vi "Create Fast Draw Object.vi"(6 "Actual Transform In":T1, 8 "error in (no error)":errorcluster, 9 "Multiplot Representation In":T3, 10 "3D Contour in":refnum<class "3D Contour.lvclass">, 11 "Plot Object In":refnum<vi>) -> (0 "error out":errorcluster, 1 "Multiplot Representation In":T3, 2 "3D Contour out":refnum<class "3D Contour.lvclass">, 3 "Plot Object Out":refnum<vi>, 4 "Actual Transform Out":T1)   [LabVIEW 2020, in "3D Contour.lvclass"]
uses:
  <vilib>/Math Plots/3D Math Plots/3D Contour/3D Contour/3D Contour.lvclass
  <vilib>/Math Plots/3D Math Plots/3D Plot/3D Plot/Typedef/Multiplot Representation.ctl
  <vilib>/Math Plots/3D Math Plots/3D Plot/3D Plot/Typedef/Plot Representation.ctl
  <vilib>/Math Plots/3D Math Plots/3D Plot/3D Plot/Typedef/Range Clusters.ctl
  <vilib>/Math Plots/3D Math Plots/3D Plot/3D Plot/Typedef/Mesh Data.ctl
  <vilib>/Math Plots/3D Math Plots/3D Plot/3D Plot/Typedef/Actual Transform.ctl
  <vilib>/Math Plots/3D Math Plots/3D Contour/3D Contour/3D Contour.lvclass/3D Contour.ctl
  <vilib>/Math Plots/3D Math Plots/3D Plot/3D Plot/3D Plot.lvclass
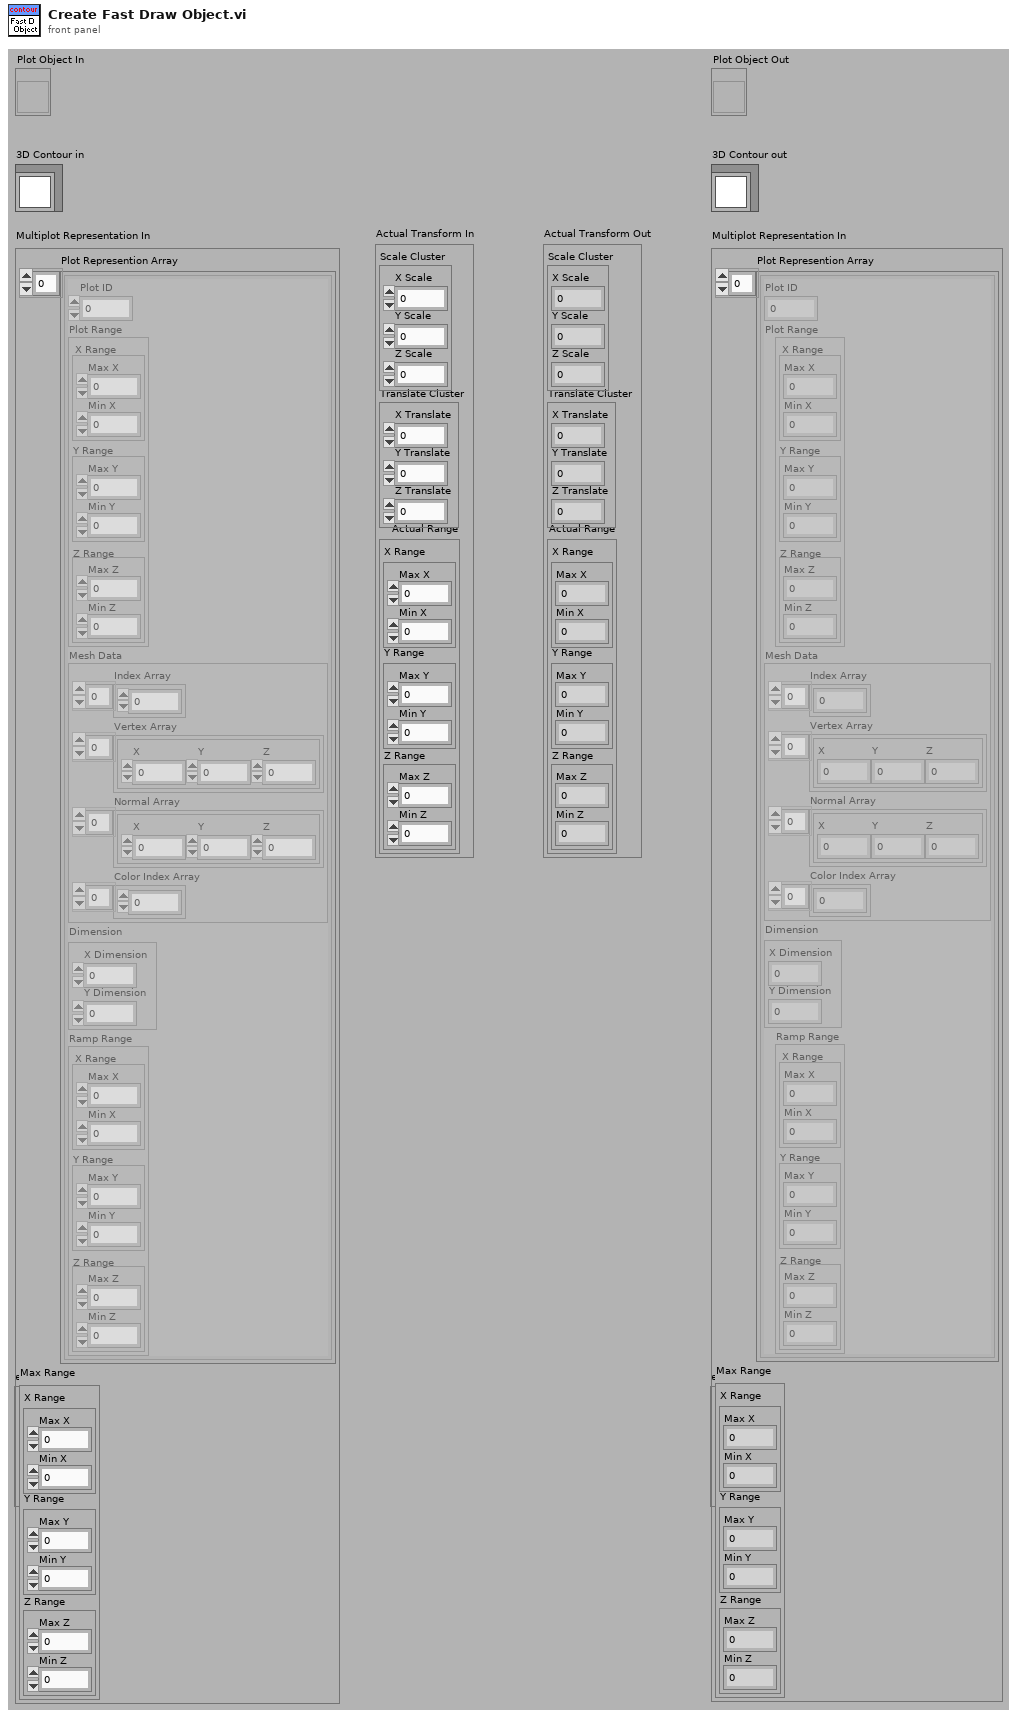
[diagram p1: front panel]
types:
  T1 = typedef "3D Plot.lvclass/Actual Transform.ctl" = cluster{"Scale Cluster":cluster{"X Scale":sgl, "Y Scale":sgl, "Z Scale":sgl}, "Translate Cluster":cluster{"X Translate":sgl, "Y Translate":sgl, "Z Translate":sgl}, "Actual Range":T2}
  T2 = typedef "3D Plot.lvclass/Range Clusters.ctl" = cluster{"X Range":cluster{"Max X":sgl, "Min X":sgl}, "Y Range":cluster{"Max Y":sgl, "Min Y":sgl}, "Z Range":cluster{"Max Z":sgl, "Min Z":sgl}}
  T3 = typedef "3D Plot.lvclass/Multiplot Representation.ctl" = cluster{"Plot Represention Array":T4[], "Max Range":T2}
  T4 = typedef "3D Plot.lvclass/Plot Representation.ctl" = cluster{"Plot ID":i32, "Plot Range":T2, "Mesh Data":T5, "Dimension":cluster{"X Dimension":i32, "Y Dimension":i32}, "Ramp Range":T2}
  T5 = typedef "3D Plot.lvclass/Mesh Data.ctl" = cluster{"Index Array":u32[], "Vertex Array":cluster{"X":sgl, "Y":sgl, "Z":sgl}[], "Normal Array":cluster{"X":sgl, "Y":sgl, "Z":sgl}[], "Color Index Array":i32[]}
  T6 = typedef "3D Contour.lvclass/3D Contour Property Array.ctl" = T7[]
  T7 = typedef "3D Contour.lvclass/3D Contour Property.ctl" = cluster{"General Property":cluster{"Plot Name":string, "Coordinate System":enum16{"Cartesian", "Cylindrical", "Spherical"}, "Opacity":sgl}, "Projection Property":cluster{"Draw XY":bool, "Draw YZ":bool, "Draw XZ":bool}, "Plot Property":cluster{"Line Style":T8, "Line Width":sgl, "Line Color":u32, "Antialiasing":bool, "Color Ramp Cluster":T9}, "Contour Property":cluster{"Contour Type":enum16{"Contour", "Contour with surface"}, "Axis Basis":enum16{"X-Axis", "Y-Axis", "Z-Axis"}, "Level List":sgl[], "Level Mode":enum16{"Levels", "Interval", "Level List"}, "Levels":u16, "Interval":sgl}}
  T8 = typedef "3D Plot.lvclass/Line Type.ctl" = enum16{"None", "Solid", "Dash", "Dot", "Dash Dot"}
  T9 = typedef "3D Plot.lvclass/Color Ramp Cluster.ctl" = cluster{"Color Ramp Style":enum16{"None", "Shaded", "Color spectrum", "Grey scale", "Custom"}, "Color Ramp Array":u32[], "Color Ramp Index":i32[], "Interpolate?":bool, "Logarithm?":bool}
  T10 = enum16{"Points", "Lines", "Line Strip", "Line Loop", "Triangles", "Triangle Strip", "Triangle Fan", "Quads", "Quad Strip", "Polygon"}
  T11 = cluster{"Draw XY":bool, "Draw YZ":bool, "Draw XZ":bool}
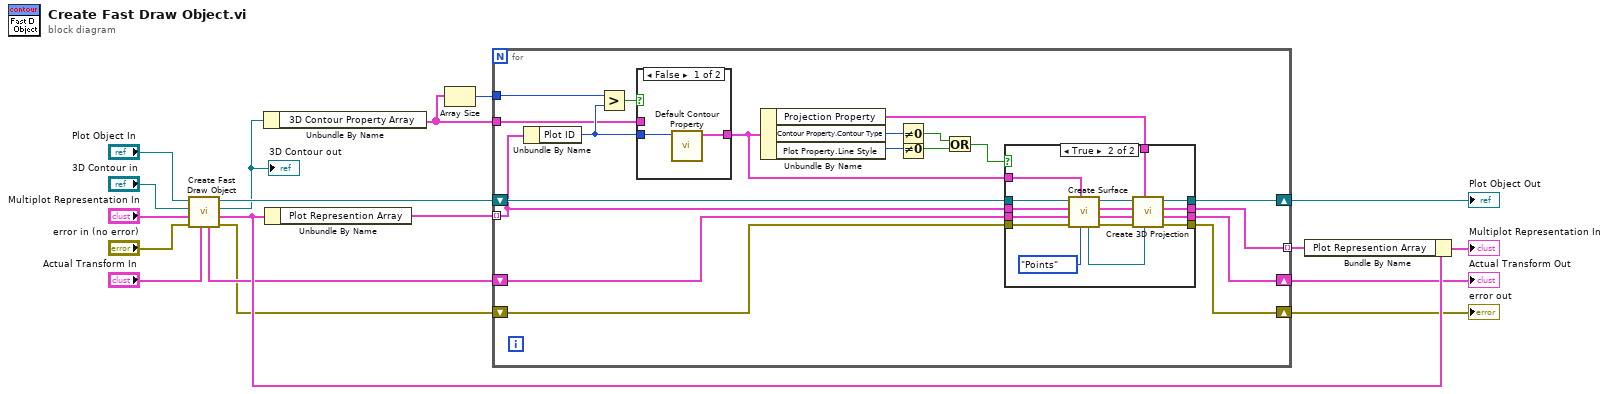
[diagram p0: block diagram]
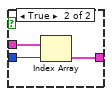
[diagram p2: hidden frame]
diagram:
  n1 = call-parent "Create Fast Draw Object.vi"("Actual Transform In"="Actual Transform In", "error in (no error)"="error in (no error)", "Multiplot Representation In"="Multiplot Representation In", "3D Plot.lvclass in"="3D Contour in", "Plot Object In"="Plot Object In") -> ("error out"=w4:errorcluster, "Multiplot Representation Out"=w11:T3, "3D Plot.lvclass out"=w3:refnum<class "3D Contour.lvclass">, "Plot Object Out"=w14:refnum<vi>, "Actual Transform Out"=w8:T1)  [unwired: 2 out]
  "3D Contour out" <- w3
  n2 = Unbundle By Name(w3) -> ("3D Contour Property Array"=w1:T6)
  n3 = Unbundle By Name(w11) -> ("Plot Represention Array"=w18:T4[])
  n4 = Array Size(array=w1) -> (size(s)=w2:i32)
  n5 = for {
    tunnel: w18 -> [w33] mode=indexing
    tunnel: [w35] -> w16 mode=indexing
    shift-right: [w31] -> w7
    shift-left: w8 -> [w34]
    shift-right: [w30] -> w6
    shift-left: w4 -> [w36]
    shift-right: [w32] -> w5
    shift-left: w14 -> [w37]
    tunnel: w1 -> [w20]
    tunnel: w2 -> [w19]
    n6 = Unbundle By Name(w33) -> ("Plot ID"=w22:i32)
    n7 = Greater?(x=w19, y=w22) -> (0:w23:bool)
    n8 = case shown="False" w23 {
      tunnel: w20 -> [_ w42]
      tunnel: [w38 w41] -> w21
      tunnel: w22 -> [w39 w40]
      frame False {
        n9 = call <vilib>:"Default Contour Property.vi"("Plot ID"=w39) -> ("Default Property"=w38:T7)  [unwired: 10 out]
      }
      frame True {
        n10 = Index Array(array=w42, index=w40) -> (element=w41:T7)
      }
    }
    n11 = Unbundle By Name(w21) -> ("Projection Property"=w29:T11, "Contour Property.Contour Type"=w28:enum16{"Contour", "Contour with surface"}, "Plot Property.Line Style"=w27:T8)
    n12 = Not Equal To 0?(x=w28) -> (x != 0?=w26:bool)
    n13 = Not Equal To 0?(x=w27) -> (x != 0?=w25:bool)
    n14 = Or(x=w26, y=w25) -> (x .or. y?=w24:bool)
    n15 = case shown="True" w24 {
      tunnel: w37 -> [w46 w61]
      tunnel: w36 -> [w43 w60]
      tunnel: [w45 w59] -> w35
      tunnel: w34 -> [w44 w58]
      tunnel: w33 -> [w45 w57]
      tunnel: [w46 w53] -> w32
      tunnel: [w44 w52] -> w31
      tunnel: [w43 w51] -> w30
      tunnel: w29 -> [_ w49]
      tunnel: w21 -> [_ w48]
      frame False {
      }
      frame True {
        n16 = call <vilib>:"Create Surface.vi"("Draw Mode"=T10."Points", "3D Contour Property"=w48, "error in (no error)"=w60, "Actual Transform In"=w58, "Plot Representation In"=w57, "Plot Object In"=w61) -> ("error out"=w54:errorcluster, "Actual Transform Out"=w55:T1, "Plot Representation Out"=w59:T4, "Plot Object Out"=w56:refnum<vi>, "Surface Object Out"=w50:refnum<vi>)  [unwired: 1 in]
        n17 = call <vilib>:"Create 3D Projection.vi"("Sub Object In"=w50, "Projection Property"=w49, "error in (no error)"=w54, "Actual Transform In"=w55, "Plot Object In"=w56) -> ("error out"=w51:errorcluster, "Actual Transform Out"=w52:T1, "Plot Object Out"=w53:refnum<vi>)  [unwired: 1 in, 3 out]
      }
    }
  }
  "error out" <- w6
  "Plot Object Out" <- w5
  "Actual Transform Out" <- w7
  n18 = Bundle By Name(cluster=w11, "Plot Represention Array"=w16) -> (→"Multiplot Representation In":T3)
